vi "Semaphore Create Acquire.vi"(7 "Timeout (ms)":u16=65535, 8 "error in":errorcluster, 9 "MaximumCount":i32=1, 10 "Initial Count":i32=1, 11 "Name":string="LabVIEW_System_Semaphore") -> (0 "error out":errorcluster, 2 "Timed Out?":bool, 3 "TDM IO Lock":u16)   [LabVIEW 2011]
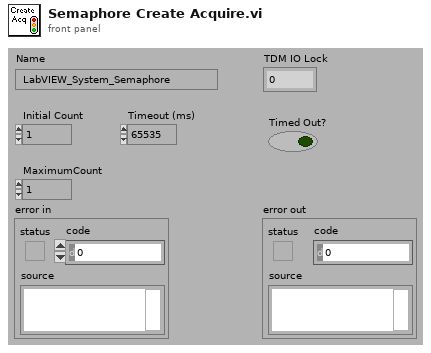
[diagram p1: front panel]
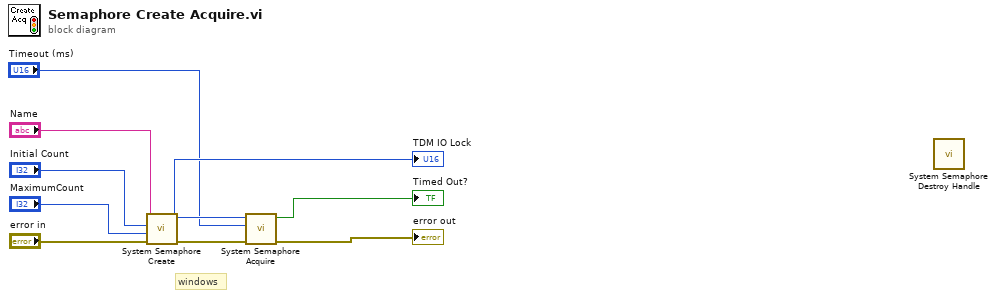
[diagram p0: block diagram]
diagram:
  # "windows"
  n1 = call "System Semaphore Create.vi"("error in (no error)"="error in", "MaximumCount"="MaximumCount", "Initial Count"="Initial Count", "Name"="Name") -> ("error out"=w1:errorcluster, "Handle"=w5:u16)  [unwired: 6 in]
  "TDM IO Lock" <- w5
  n2 = call "System Semaphore Acquire.vi"("error in (no error)"=w1, "Timeout (ms)"="Timeout (ms)", "SemaphoreHandle"=w5) -> ("error out"=→"error out":errorcluster, "Timed Out?"=→"Timed Out?":bool)  [unwired: 6 in, 1 out]
  n3 = call "System Semaphore Destroy Handle.vi"() -> ()  [unwired: 11 in, 1 out]
